vi "S2C_ExeScriptPassResultRoute.vi"(8 "Error In":errorcluster, 10 "LastStep?":bool, 11 "Q_Ref":refnum<queue>) -> (0 "Error Out":errorcluster, 3 "IncRow?":bool)   [LabVIEW 2015]
doc: "Update the results cell in the execution table for the currently executing line item, and determines the next step to take in the execution."
uses:
  Controls/S2C_ExePause.ctl
  Globals/S2C_Globals.vi
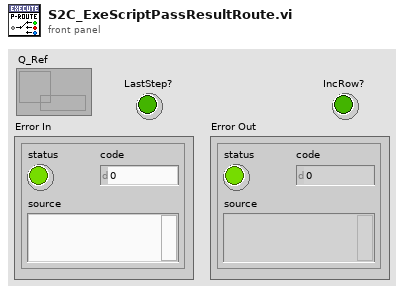
[diagram p1: front panel]
types:
  T1 = typedef "S2C_ExePause.ctl" = bool
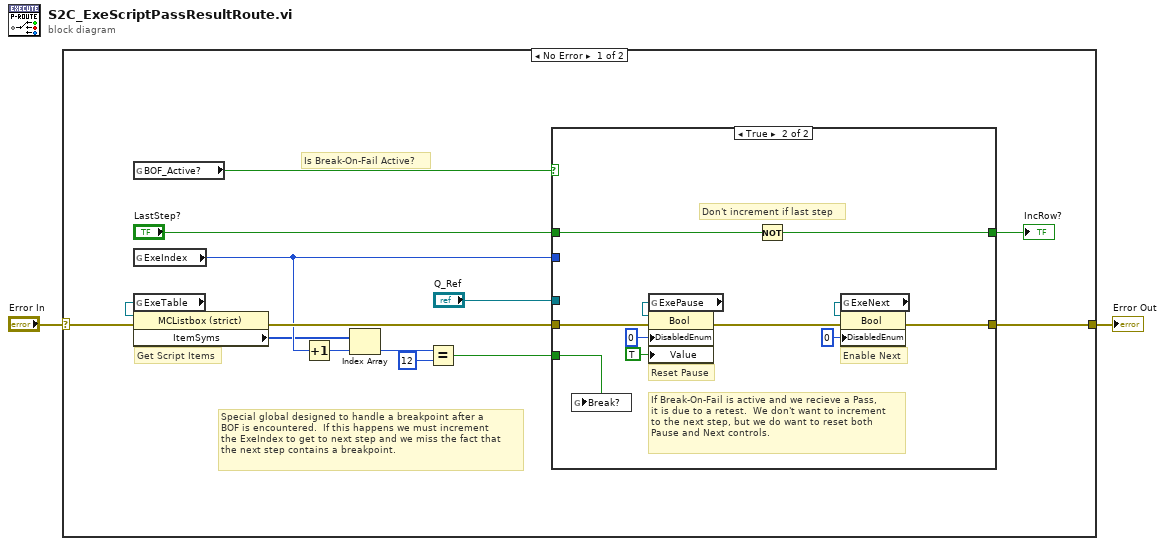
[diagram p0: block diagram]
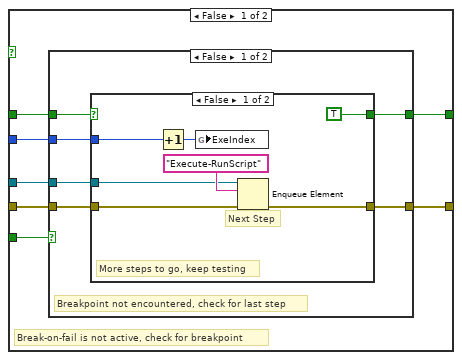
[diagram p2: hidden frame]
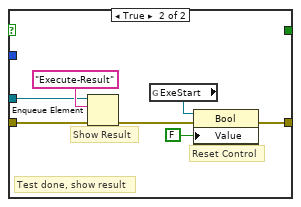
[diagram p3: hidden frame]
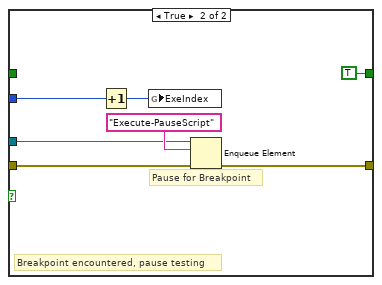
[diagram p4: hidden frame]
diagram:
  n1 = case shown="No Error" "Error In" {
    selector: "Error In" -> [w12 w62]
    tunnel: [w15 w62] -> w1
    frame No Error {
      # "Special global designed to handle a breakpoint after a\nBOF is encountered.  If this happens we must increment\nthe ExeIndex to get to next step and we miss the fact that\nthe next step contains a breakpoint."
      # "Is Break-On-Fail Active?"
      # "Get Script Items"
      n2 = global read "S2C_Globals.vi" "BOF_Active?"() -> (w10:bool)
      n3 = global read "S2C_Globals.vi" "ExeIndex"() -> (w5:i32)
      n4 = global read "S2C_Globals.vi" "ExeTable"() -> (w13:refnum<vi>)
      n5 = property class="MCListbox (strict)"(reference=w13, error in=w12) -> (error out=w11:errorcluster, "ItemSyms"=w4:i32[])  [unwired: 1 out]
      n6 = Increment(x=w5) -> (x+1=w8:i32)
      n7 = Index Array(array=w4, index=w8) -> (element=w6:i32)
      n8 = Equal?(x=w6, y=12) -> (x = y?=w3:bool)
      n9 = case shown="True" w10 {
        tunnel: "Q_Ref" -> [w23 _]
        tunnel: [w22 w54] -> w15
        tunnel: "LastStep?" -> [w21 w53]
        tunnel: w5 -> [w20 _]
        tunnel: w11 -> [w19 w55]
        tunnel: w3 -> [w18 w51]
        tunnel: [w17 w52] -> w9
        frame False {
          # "Break-on-fail is not active, check for breakpoint"
          n10 = case shown="False" w18 {
            tunnel: w20 -> [w27 w46]
            tunnel: w19 -> [w29 w49]
            tunnel: [w28 w48] -> w22
            tunnel: w23 -> [w26 w47]
            tunnel: w21 -> [w25 _]
            tunnel: [w24 TRUE] -> w17
            frame False {
              # "Breakpoint not encountered, check for last step"
              n11 = case shown="False" w25 {
                tunnel: w29 -> [w36 w39]
                tunnel: [w35 w37] -> w28
                tunnel: w27 -> [w32 _]
                tunnel: w26 -> [w31 w38]
                tunnel: [TRUE _] -> w24
                frame False {
                  # "More steps to go, keep testing"
                  # "Next Step"
                  n12 = Increment(x=w32) -> (x+1=w33:i32)
                  n13 = global write "S2C_Globals.vi" "ExeIndex"(w33) -> ()
                  n14 = Enqueue Element(queue=w31, element="Execute-RunScript", error in (no error)=w36) -> (error out=w35:errorcluster)  [unwired: 1 in, 2 out]
                }
                frame True {
                  # "Test done, show result"
                  # "Show Result"
                  # "Reset Control"
                  n15 = Enqueue Element(queue=w38, element="Execute-Result", error in (no error)=w39) -> (error out=w41:errorcluster)  [unwired: 1 in, 2 out]
                  n16 = global read "S2C_Globals.vi" "ExeStart"() -> (w43:refnum<vi>)
                  n17 = property class="Bool"(reference=w43, error in=w41, "Value"=FALSE) -> (error out=w37:errorcluster)  [unwired: 1 out]
                }
              }
            }
            frame True {
              # "Breakpoint encountered, pause testing"
              # "Pause for Breakpoint"
              n18 = Increment(x=w46) -> (x+1=w44:i32)
              n19 = global write "S2C_Globals.vi" "ExeIndex"(w44) -> ()
              n20 = Enqueue Element(queue=w47, element="Execute-PauseScript", error in (no error)=w49) -> (error out=w48:errorcluster)  [unwired: 1 in, 2 out]
            }
          }
        }
        frame True {
          # "Don't increment if last step"
          # "If Break-On-Fail is active and we recieve a Pass,\nit is due to a retest.  We don't want to increment\nto the next step, but we do want to reset both\nPause and Next controls."
          # "Enable Next"
          # "Reset Pause"
          n21 = global write "S2C_Globals.vi" "Break?"(w51) -> ()
          n22 = global read "S2C_Globals.vi" "ExePause"() -> (w59:refnum<vi>)
          n23 = property on="Property Node" class="Bool"(reference=w59, error in=w55, "DisabledEnum"=u8 0, "Value"=T1 TRUE) -> (error out=w56:errorcluster)  [unwired: 1 out]
          n24 = Not(x=w53) -> (.not. x?=w52:bool)
          n25 = global read "S2C_Globals.vi" "ExeNext"() -> (w57:refnum<vi>)
          n26 = property on="Property Node" class="Bool"(reference=w57, error in=w56, "DisabledEnum"=u8 0) -> (error out=w54:errorcluster)  [unwired: 1 out]
        }
      }
      "IncRow?" <- w9
    }
    frame Error {
    }
  }
  "Error Out" <- w1
